vi "Close.vi"(8 "error in (no error)":errorcluster, 11 "Cryo Cooler in":refnum<class "Cryo Cooler.lvclass">) -> (0 "error out":errorcluster, 3 "Cryo Cooler out":refnum<class "Cryo Cooler.lvclass">)   [LabVIEW 2024, in "Cryo Cooler.lvclass"]
uses:
  Cryo Cooler.lvclass
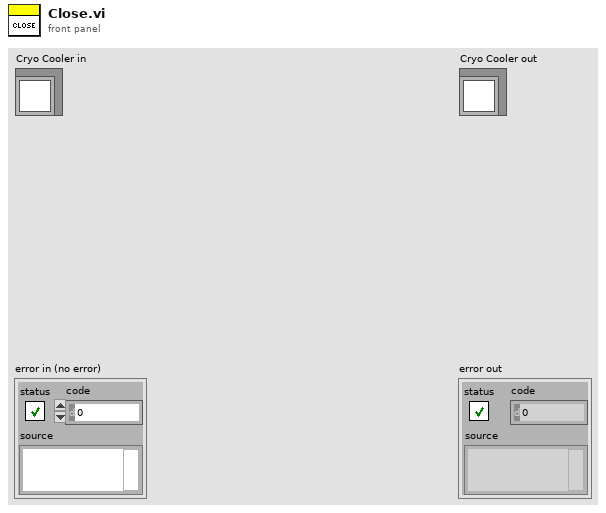
[diagram p1: front panel]
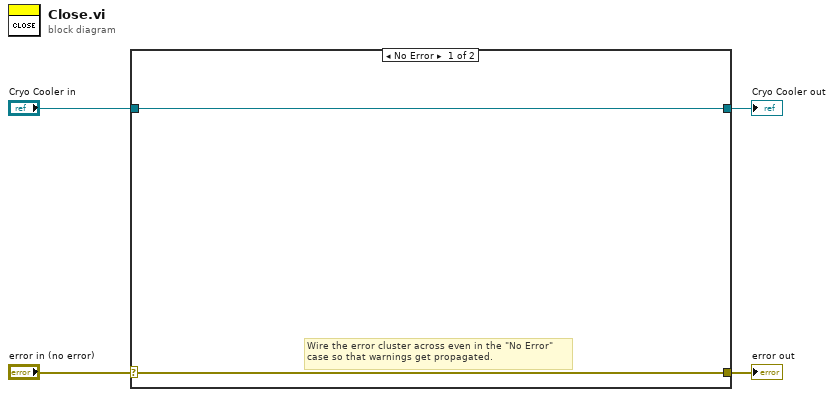
[diagram p0: block diagram]
diagram:
  n1 = case shown="No Error" "error in (no error)" {
    selector: "error in (no error)" -> [w5 w8]
    tunnel: [w5 w8] -> w3
    tunnel: [w6 w7] -> w1
    tunnel: "Cryo Cooler in" -> [w6 w7]
    frame No Error {
      # "Wire the error cluster across even in the \"No Error\"\ncase so that warnings get propagated."
    }
    frame Error {
    }
  }
  "error out" <- w3
  "Cryo Cooler out" <- w1
